vi "Coherence_Fit_Test.vi"() -> ()   [LabVIEW 2020]
doc: "Attempt to fit a decaying exponential to computed FFT of LLM data\n\nSlope of dacaying exponential should give you the coherence time for the laser\n\nR. Sheehan 11 - 11 - 2021"
uses:
  <vilib>/Utility/file.llb/Read Delimited Spreadsheet (DBL).vi
  <vilib>/Analysis/NI_AALPro.lvlib
panel:
  out "tauc / ns":dbl=51.7318662762112
  out "intercept":dbl=7.817821381057423
  out "slope":dbl=-19.33044508119453
  out "XY Graph 3":T1(graph)=[{"all rows"=array[4096 elements], "Best Linear Fit"=array[4096 elements]}, {"all rows"=[0.0, 0.01953601954, 0.03907203907, 0.05860805861, 0.07814407814, 0.09768009768, 0.1172161172, 0.1367521368, 0.1562881563, 0.1758241758, 0.1953601954, 0.2148962149, 0.2344322344, 0.253968254, 0.2735042735, 0.293040293, 0.3125763126, 0.3321123321, 0.3516483516, 0.3711843712, 0.3907203907], "Best Linear Fit"=[7.11356342629216, 6.994156940049452, 6.796026501587647, 6.640349594656045, 6.4007592001397065, 6.147711251098183, 5.893261755106928, 5.5588709592768595, 5.262777736885921, 4.883447957800071, 4.46139480054909, 4.092742154719343, 3.465064458994278, 3.052824384807083, 2.3490679650300326, 1.5288289208020647, 1.4985585007580957, 1.1752181926764387, 0.6387506181183747, -0.23823702574886, 1.154720632377344]}, {"all rows"=[0.0, 0.01953601954, 0.03907203907, 0.05860805861, 0.07814407814, 0.09768009768, 0.1172161172, 0.1367521368, 0.1562881563, 0.1758241758, 0.1953601954, 0.2148962149, 0.2344322344, 0.253968254, 0.2735042735, 0.293040293, 0.3125763126, 0.3321123321, 0.3516483516, 0.3711843712, 0.3907203907], "Best Linear Fit"=[7.817821381057423, 7.44018142823431, 7.062541475604501, 6.684901522781388, 6.30726157015158, 5.929621617328467, 5.5519816648919615, 5.174341710909022, 4.796701758859126, 4.419061806809231, 4.041421852826291, 3.663781900776396, 3.2861419487265007, 2.9085019947435606, 2.5308620426936645, 2.1532220906437693, 1.7755821366608293, 1.3979421846109341, 1.020302232561039, 0.6426622785780998, 0.2650223265282037]}]
  out "XY Graph 2":cluster{"all rows":dbl[], "all rows":dbl[]}(graph)
  out "XY Graph":cluster{"all rows":dbl[], "all rows":dbl[]}(graph)
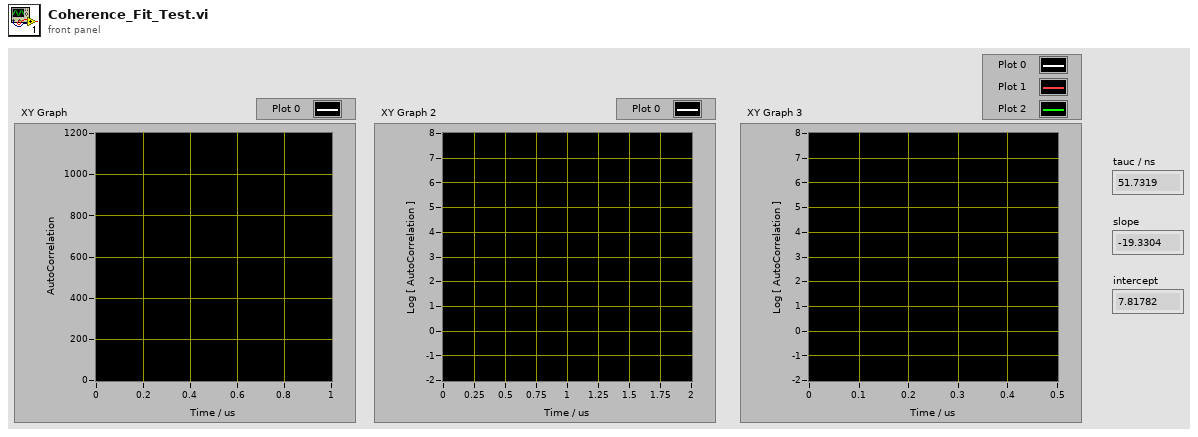
[diagram p1: front panel]
types:
  T1 = cluster{"all rows":dbl[], "Best Linear Fit":dbl[]}[]
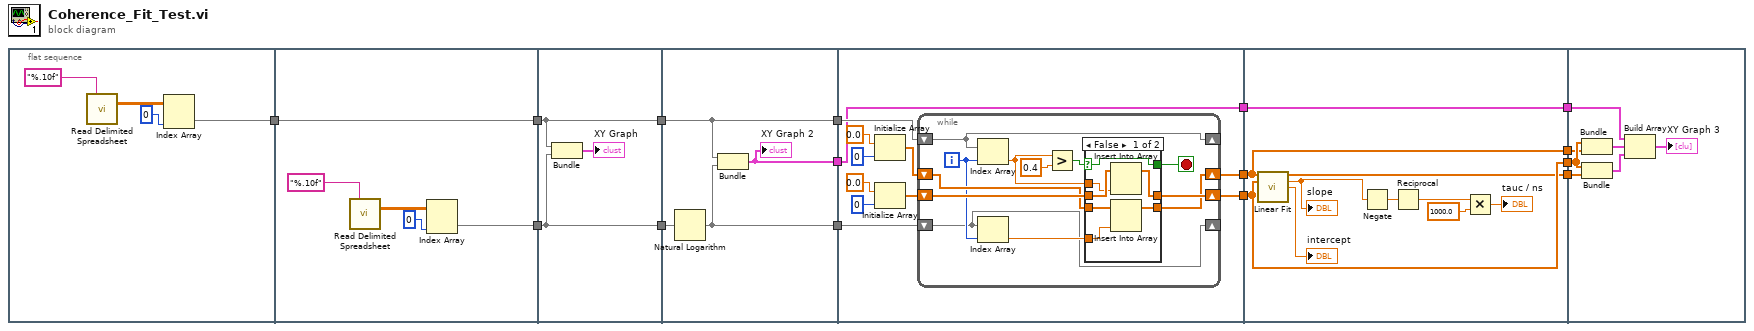
[diagram p0: block diagram]
diagram:
  n1 = flat-sequence {
    tunnel: [w16] -> w14
    tunnel: [w21] -> w15
    tunnel: w14 -> [w21]
    tunnel: [w20] -> w13
    tunnel: w15 -> [w25]
    tunnel: w13 -> [w26]
    tunnel: [w26] -> w12
    tunnel: [w25] -> w11
    tunnel: w12 -> [w31]
    tunnel: w11 -> [w30]
    tunnel: [w30] -> w10
    tunnel: [w29] -> w9
    tunnel: [w28] -> w1
    tunnel: w10 -> [w42]
    tunnel: w9 -> [w35]
    tunnel: [w34] -> w8
    tunnel: [w33] -> w7
    tunnel: [w32] -> w2
    tunnel: w1 -> [w32]
    tunnel: w8 -> [w72]
    tunnel: w7 -> [w74]
    tunnel: [w74] -> w6
    tunnel: [w73] -> w5
    tunnel: [w72] -> w4
    tunnel: [w71] -> w3
    tunnel: w2 -> [w71]
    tunnel: w6 -> [w80]
    tunnel: w5 -> [w81]
    tunnel: w4 -> [w79]
    tunnel: w3 -> [w76]
    frame #0 {
      n2 = call-poly <vilib>:"Read Delimited Spreadsheet.vi"("format (%.3f)"="%.10f") -> ("all rows"=w18:dbl[][])  [unwired: 9 in, 5 out]
      n3 = Index Array(array=w18, index (col)=0 ("disabled index (col)")) -> (element=w16:dbl[])  [unwired: 1 in]
    }
    frame #1 {
      n4 = call-poly <vilib>:"Read Delimited Spreadsheet.vi"("format (%.3f)"="%.10f") -> ("all rows"=w23:dbl[][])  [unwired: 9 in, 5 out]
      n5 = Index Array(array=w23, index (col)=0 ("disabled index (col)")) -> (element=w20:dbl[])  [unwired: 1 in]
    }
    frame #2 {
      n6 = Bundle("all rows"=w25, "all rows"=w26) -> (→"XY Graph":cluster{"all rows":dbl[], "all rows":dbl[]})  [unwired: 1 in]
    }
    frame #3 {
      n7 = Natural Logarithm(1:w31) -> (0:w29:dbl[])
      n8 = Bundle("all rows"=w30, w29) -> (w28:cluster{"all rows":dbl[], dbl[]})  [unwired: 1 in]
      "XY Graph 2" <- w28
    }
    frame #4 {
      n9 = Initialize Array(0.0 ("element"), 0 ("dimension size")) -> (w36:dbl[])
      n10 = Initialize Array(0.0 ("element"), 0 ("dimension size")) -> (w37:dbl[])
      n11 = while {
        shift-right: [w46] -> _
        shift-left: w42 -> [w46]
        shift-right: [w52] -> w33
        shift-left: w37 -> [w53]
        shift-right: [w50] -> w34
        shift-left: w36 -> [w51]
        shift-right: [w43] -> _
        shift-left: w35 -> [w43]
        i -> [w45]
        stop <- w48 stop-if-true
        n12 = Index Array(array=w46, index=w45) -> (element=w47:dbl)
        n13 = Index Array(array=w43, index=w45) -> (element=w44:dbl)
        n14 = Greater?(x=w47, y=0.4) -> (0:w49:bool)
        n15 = case shown="False" w49 {
          selector: w49 -> [w57 w62]
          tunnel: w53 -> [w61 w64]
          tunnel: [w60 w64] -> w52
          tunnel: w51 -> [w59 w63]
          tunnel: [w58 w63] -> w50
          tunnel: [w57 w62] -> w48
          tunnel: w47 -> [w56 _]
          tunnel: w44 -> [w55 _]
          frame False {
            n16 = Insert Into Array(array=w61, new element=w56) -> (w60:dbl[])  [unwired: 1 in]
            n17 = Insert Into Array(array=w59, new element=w55) -> (w58:dbl[])  [unwired: 1 in]
          }
          frame True {
          }
        }
      }
    }
    frame #5 {
      n18 = call <vilib>:"Linear Fit.vi"("Y"=w72, "X"=w74) -> ("Best Linear Fit"=w73:dbl[], "slope"=w69:dbl, "intercept"=→"intercept":dbl)  [unwired: 9 in, 2 out]
      "slope" <- w69
      n19 = Negate(x=w69) -> (-x=w68:dbl)
      n20 = Reciprocal(x=w68) -> (1/x=w67:dbl)
      n21 = Multiply(x=w67, y=1000.0) -> (x*y=→"tauc / ns":dbl)
    }
    frame #6 {
      n22 = Bundle(w80, w79) -> (w78:cluster{dbl[], dbl[]})  [unwired: 1 in]
      n23 = Bundle(w80, "Best Linear Fit"=w81) -> (w77:cluster{dbl[], "Best Linear Fit":dbl[]})  [unwired: 1 in]
      n24 = Build Array(w76, w78, w77) -> (→"XY Graph 3":T1)
    }
  }
